vi "Cal Attendance.vi"(8 "error in (no error)":errorcluster, 11 "MemberAttendance in":refnum<class "MemberAttendance.lvclass">) -> (0 "error out":errorcluster, 2 "Attendance Result(\"\")":string[][](array[string]), 3 "MemberAttendance out":refnum<class "MemberAttendance.lvclass">)   [LabVIEW 2015, in "Admin_Actor.lvlib" / "MemberAttendance.lvclass"]
uses:
  MemberAttendance.lvclass
  MemberAttendance.lvclass/MemberAttendance.ctl
  Setting/g_setting.vi
  Admin_Actor.lvlib
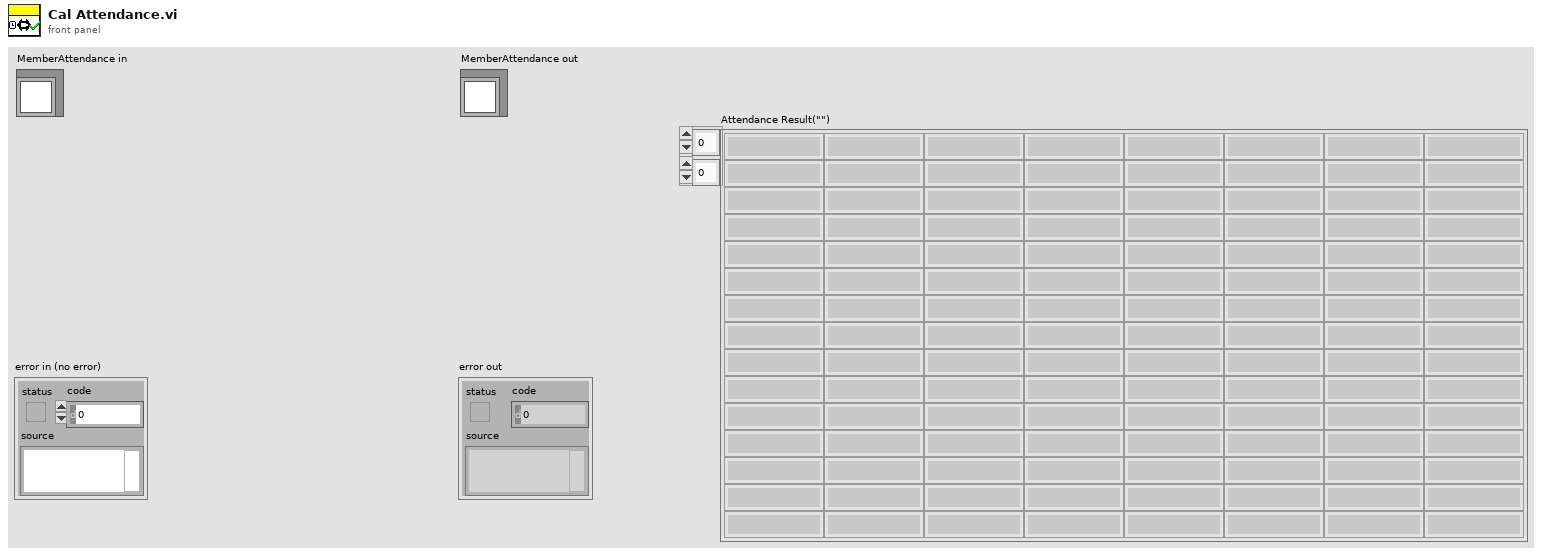
[diagram p1: front panel]
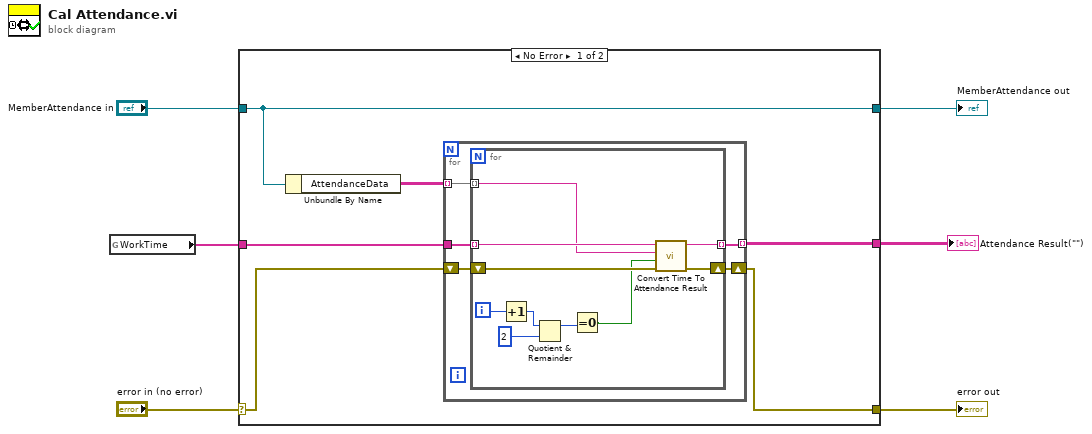
[diagram p0: block diagram]
diagram:
  n1 = global read "g_setting.vi" "WorkTime"() -> (w2:string[])
  n2 = case shown="No Error" "error in (no error)" {
    selector: "error in (no error)" -> [w10 w29]
    tunnel: [w9 w29] -> w5
    tunnel: [w7 w28] -> w3
    tunnel: "MemberAttendance in" -> [w7 w28]
    tunnel: w2 -> [w11 _]
    tunnel: [w8 _] -> w1
    frame No Error {
      n3 = Unbundle By Name(w7) -> ("AttendanceData"=w12:string[][])
      n4 = for {
        tunnel: w12 -> [w17] mode=indexing
        tunnel: w11 -> [w16]
        shift-right: [w14] -> w9
        shift-left: w10 -> [w15]
        tunnel: [w13] -> w8 mode=indexing
        n5 = for {
          tunnel: w17 -> [w26] mode=indexing
          tunnel: w16 -> [w27] mode=indexing
          shift-right: [w22] -> w14
          shift-left: w15 -> [w23]
          tunnel: [w21] -> w13 mode=indexing
          i -> [w20]
          n6 = Increment(x=w20) -> (x+1=w19:i32)
          n7 = Quotient & Remainder(x=w19, y=2) -> (x-y*floor(x/y)=w24:i32)  [unwired: 1 out]
          n8 = Equal To 0?(x=w24) -> (x = 0?=w18:bool)
          n9 = call "Convert Time To Attendance Result.vi"("error in (no error)"=w23, "上班/下班（上班）"=w18, "ActualTime(\"\")"=w26, "StandardTime(\"\")"=w27) -> ("error out"=w22:errorcluster, "Actual Circustance"=w21:string)  [unwired: 6 in]
        }
      }
    }
    frame Error {
    }
  }
  "error out" <- w5
  "MemberAttendance out" <- w3
  "Attendance Result(\"\")" <- w1
